vi "Set Active Program.vi"(8 "error in (no error)":errorcluster, 10 "Scene Name":string, 11 "OBS in":refnum<class "OBS.lvclass">) -> (0 "error out":errorcluster, 3 "OBS out":refnum<class "OBS.lvclass">)   [LabVIEW 2022 SP3, in "obs-websocket-lv.lvlib" / "OBS.lvclass"]
uses:
  OBS.lvclass
  OBS.lvclass/OBS.ctl
  SetCurrentProgramScene/SetCurrentProgramScene.lvclass
  C:/dev/illuminatedg/obs-websocket-lv/obs-websocket-lv/Request/Request.lvclass
  C:/dev/illuminatedg/obs-websocket-lv/obs-websocket-lv/Client Message/Client Message.lvclass
  C:/dev/illuminatedg/obs-websocket-lv/obs-websocket-lv/Message/Message.lvclass
  C:/dev/illuminatedg/obs-websocket-lv/obs-websocket-lv/SetCurrentProgramScene/SetCurrentProgramScene.lvclass
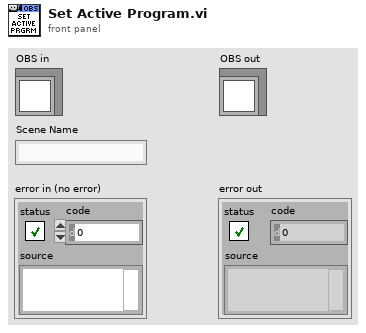
[diagram p1: front panel]
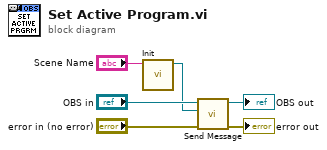
[diagram p0: block diagram]
diagram:
  n1 = call "Init.vi"("Scene Name"="Scene Name") -> ("SetCurrentProgramScene out"=w3:refnum<class "SetCurrentProgramScene.lvclass">)  [unwired: 9 in, 1 out]
  n2 = call "Send Message.vi"("error in (no error)"="error in (no error)", "Client Message"=w3, "OBS in"="OBS in") -> ("error out"=→"error out":errorcluster, "OBS out"=→"OBS out":refnum<class "OBS.lvclass">)  [unwired: 5 in, 2 out]
